vi "_StrTable to LogicCfg.vi"(8 "error in (no error)":errorcluster, 11 "CfgTable in":string[][](array[string])) -> (0 "error out":errorcluster, 3 "Array 2":T1[](array[typedef]))   [LabVIEW 2017, in "TagDB UIStateExpression.lvlib"]
uses:
  TagDB UIStateExpression.lvlib
  RefManager/Typedef/RefMgr-Logic-State.ctl
  RefManager/Typedef/RefMgr-StateChangeType.ctl
  627ab74d-fd43-4f3b-ae31-bc93842384ce.vi
  480c0bf6-53d7-4c76-b845-d201bd49c9a1.vi
  <userlib>/_OpenG.lib/string/string.llb/Trim Whitespace (String Array)__ogtk.vi
  <userlib>/NEVSTOP-Programming-Palette/Configuration/ClusterCfgTable/Parse CfgTable(with DataName).vi
  RefManager/TagDB RefManager.lvlib
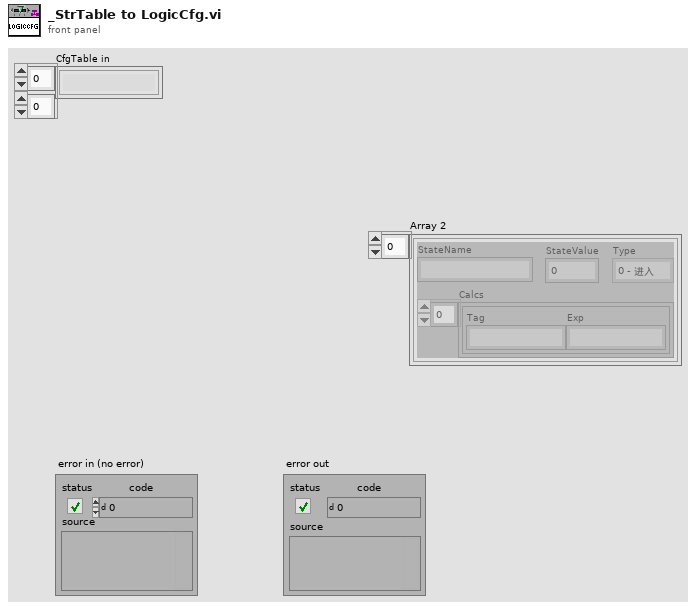
[diagram p1: front panel]
types:
  T1 = typedef "TagDB RefManager.lvlib/RefMgr-Logic-State.ctl" = cluster{"StateName":string, "StateValue":i32, "Type":T2, "Calcs":cluster{"Tag":string, "Exp":string}[]}
  T2 = typedef "TagDB RefManager.lvlib/RefMgr-StateChangeType.ctl" = enum16{"0 - 进入", "1 - 等于", "2 - 退出"}
  T3 = cluster{"StateName":string, "StateName 2":string, "StateValue":i32, "Type":T2}
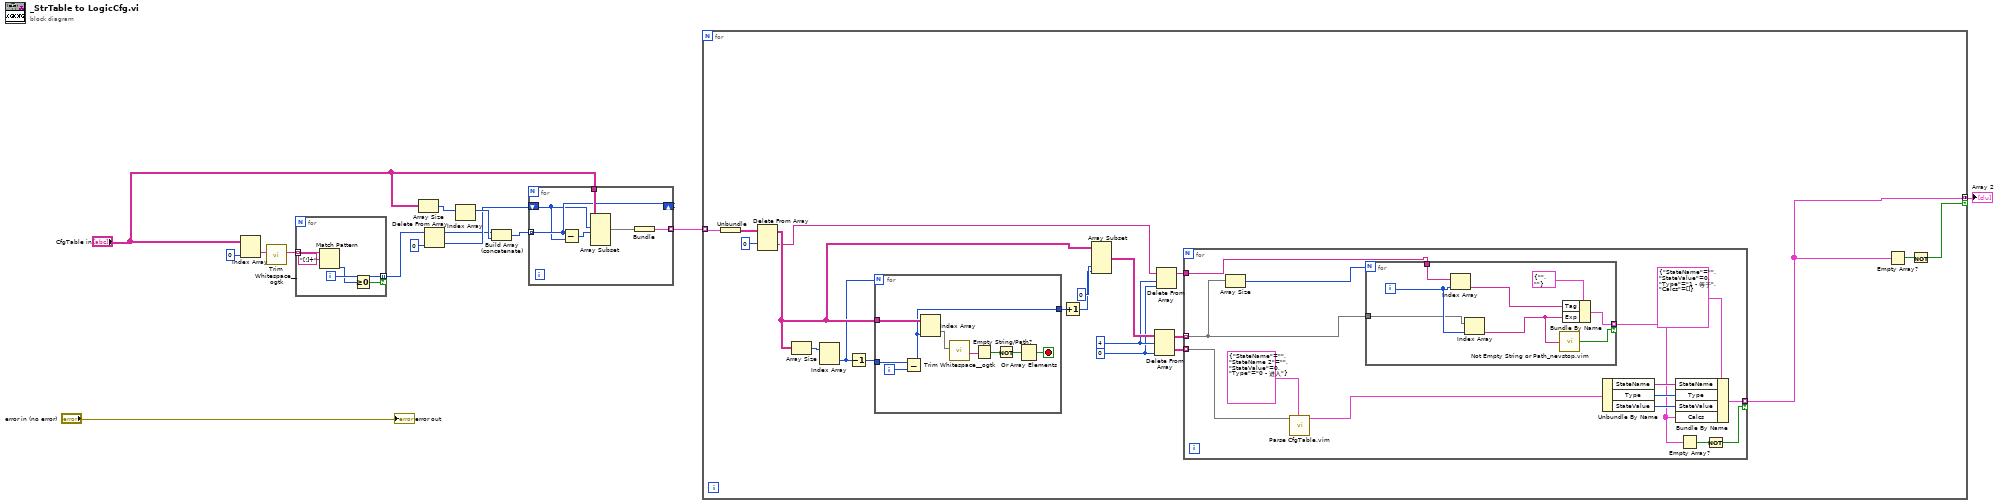
[diagram p0: block diagram]
diagram:
  n1 = Index Array(array="CfgTable in", index (col)=0 ("disabled index (col)")) -> (element=w4:string[])  [unwired: 1 in]
  n2 = call-poly <userlib>:"Trim Whitespace__ogtk.vi"("String in"=w4) -> ("String out"=w6:string[])  [unwired: 6 in]
  n3 = for {
    tunnel: w6 -> [w19] mode=indexing
    tunnel: [w17] -> w7 mode=indexing if=w15
    i -> [w17]
    n4 = Match Pattern(string=w19, regular expression="[!]+") -> (offset past match=w16:i32)  [unwired: 1 in, 3 out]
    n5 = Greater Or Equal To 0?(x=w16) -> (x >= 0?=w15:bool)
  }
  n6 = Array Size(array="CfgTable in") -> (size(s)=w12:i32[])
  n7 = Delete From Array(array=w7, index=0) -> (deleted portion=w10:i32, array with subset deleted=w9:i32[])  [unwired: 1 in]
  n8 = Index Array(array=w12) -> (element=w13:i32)  [unwired: 1 in]
  n9 = Build Array (concatenate)(w9, w13) -> (w11:i32[])
  n10 = for {
    tunnel: "CfgTable in" -> [w25]
    tunnel: w11 -> [w22] mode=indexing
    tunnel: [w23] -> w8 mode=indexing
    shift-right: [w22] -> _
    shift-left: w10 -> [w20]
    n11 = Subtract(x=w22, y=w20) -> (x-y=w21:i32)
    n12 = Array Subset(array=w25, index (row)=w20, length (row)=w21) -> (w24:string[][])  [unwired: 2 in]
    n13 = Bundle(w24) -> (w23:cluster{string[][]})  [unwired: 1 in]
  }
  n14 = for {
    tunnel: w8 -> [w45] mode=indexing
    tunnel: [w27] -> w1 mode=concatenating if=w26
    w29 = 0 ("disabled index (col)")
    w30 = 4 ("length")
    n15 = Unbundle(w45) -> (w44:string[][])
    n16 = Delete From Array(array=w44, index (row)=0 ("disabled index (col)")) -> (deleted portion=w32:string[], array with subset deleted=w40:string[][])  [unwired: 2 in]
    n17 = Array Size(array=w40) -> (size(s)=w42:i32[])
    n18 = Index Array(array=w42) -> (element #2=w37:i32)  [unwired: 2 in, 1 out]
    n19 = Decrement(x=w37) -> (x-1=w41:i32)
    n20 = for {
      N: w37 -> [_]
      tunnel: w40 -> [w76]
      tunnel: w41 -> [w75]
      tunnel: [w69] -> w39
      i -> [w70]
      stop <- w71 stop-if-true
      n21 = Subtract(x=w75, y=w70) -> (x-y=w69:i32)
      n22 = Index Array(array=w76, index (col)=w69) -> (element=w74:string[])  [unwired: 1 in]
      n23 = call-poly <userlib>:"Trim Whitespace__ogtk.vi"("String in"=w74) -> ("String out"=w73:string[])  [unwired: 6 in]
      n24 = Empty String/Path?(string/path=w73) -> (empty?=w72:bool[])
      n25 = Not(x=w72) -> (.not. x?=w68:bool[])
      n26 = Or Array Elements(Boolean array=w68) -> (logical OR=w71:bool)
    }
    n27 = Increment(x=w39) -> (x+1=w36:i32)
    n28 = Array Subset(array=w40, index (col)=0 ("index"), length (col)=w36) -> (w35:string[][])  [unwired: 2 in]
    n29 = Delete From Array(array=w35, length=w30, index (col)=w29) -> (deleted portion=w34:string[][], array with subset deleted=w33:string[][])  [unwired: 1 in]
    n30 = Delete From Array(array=w32, length=w30, index=w29) -> (array with subset deleted=w31:string[])  [unwired: 1 out]
    n31 = for {
      tunnel: w34 -> [w59] mode=indexing
      tunnel: w33 -> [w53] mode=indexing
      tunnel: w31 -> [w52]
      tunnel: [w51] -> w27 mode=indexing if=w46
      n32 = Array Size(array=w53) -> (size(s)=w48:i32)
      n33 = call "Parse CfgTable.vim"("Cluster Configuration Typedef"=T3 {"StateName"="", "StateName 2"="", "StateValue"=0, "Type"=enum."0 - 进入"} ("Cluster"), "CfgTable Row"=w59) -> ("Cluster Configuration Out"=w57:T3)  [unwired: 8 in, 1 out]
      n34 = for {
        N: w48 -> [_]
        tunnel: w53 -> [w61]
        tunnel: w52 -> [w67]
        tunnel: [w64] -> w50 mode=indexing if=w63
        i -> [w62]
        n35 = Index Array(array=w67, index=w62) -> (element=w65:string)
        n36 = Index Array(array=w61, index=w62) -> (element=w60:string)
        n37 = call "Not Empty String or Path_nevstop.vim"("String"=w60) -> ("not empty?"=w63:bool)
        n38 = Bundle By Name(cluster=cluster{"Tag":string, "Exp":string} {"Tag"="", "Exp"=""} ("Cluster"), "Tag"=w65, "Exp"=w60) -> (w64:cluster{"Tag":string, "Exp":string})
      }
      n39 = Unbundle By Name(w57) -> ("StateName"=w54:string, "Type"=w55:T2, "StateValue"=w56:i32)
      n40 = Bundle By Name(cluster=T1 {"StateName"="", "StateValue"=0, "Type"=enum."1 - 等于", "Calcs"=[]} ("Cluster"), "StateName"=w54, "Type"=w55, "StateValue"=w56, "Calcs"=w50) -> (w51:T1)
      n41 = Empty Array?(array=w50) -> (empty?=w49:bool)
      n42 = Not(x=w49) -> (.not. x?=w46:bool)
    }
    n43 = Empty Array?(array=w27) -> (empty?=w28:bool)
    n44 = Not(x=w28) -> (.not. x?=w26:bool)
  }
  "Array 2" <- w1
  "error out" <- "error in (no error)"
